vi "BIN-date2yearNum.vi"(2 "Time":timestamp) -> (7 "YearNum":u64)   [LabVIEW 2020, in "Sgraph_lib_V1.lvlib" / "DBAL-BIN.lvclass"]
doc: "Convert date to Year numerical value"
uses:
  DBAL-BIN.lvclass
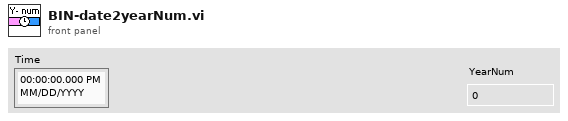
[diagram p1: front panel]
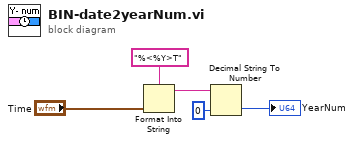
[diagram p0: block diagram]
diagram:
  n1 = Format Into String(format string="%<%Y>T", "Time") -> (resulting string=w4:string)  [unwired: 2 in, 1 out]
  n2 = Decimal String To Number(string=w4, default (0L)=u64 0 ("default (0 I32)")) -> (number=→"YearNum":u64)  [unwired: 1 in, 1 out]
